vi "regulator1.vi"(0 "histereza":dbl, 4 "H2 [cm]":dbl, 5 "H1 [cm]":dbl, 6 "h2max":dbl, 7 "h2min":dbl, 8 "h1max":dbl, 9 "h1min":dbl) -> (1 "Zawor2":bool, 2 "Zawor1":bool, 3 "Pompa":bool)   [LabVIEW 2020]
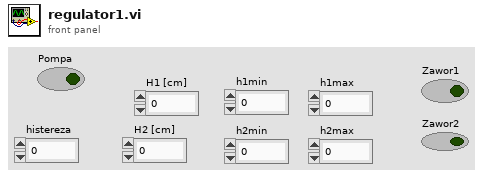
[diagram p1: front panel]
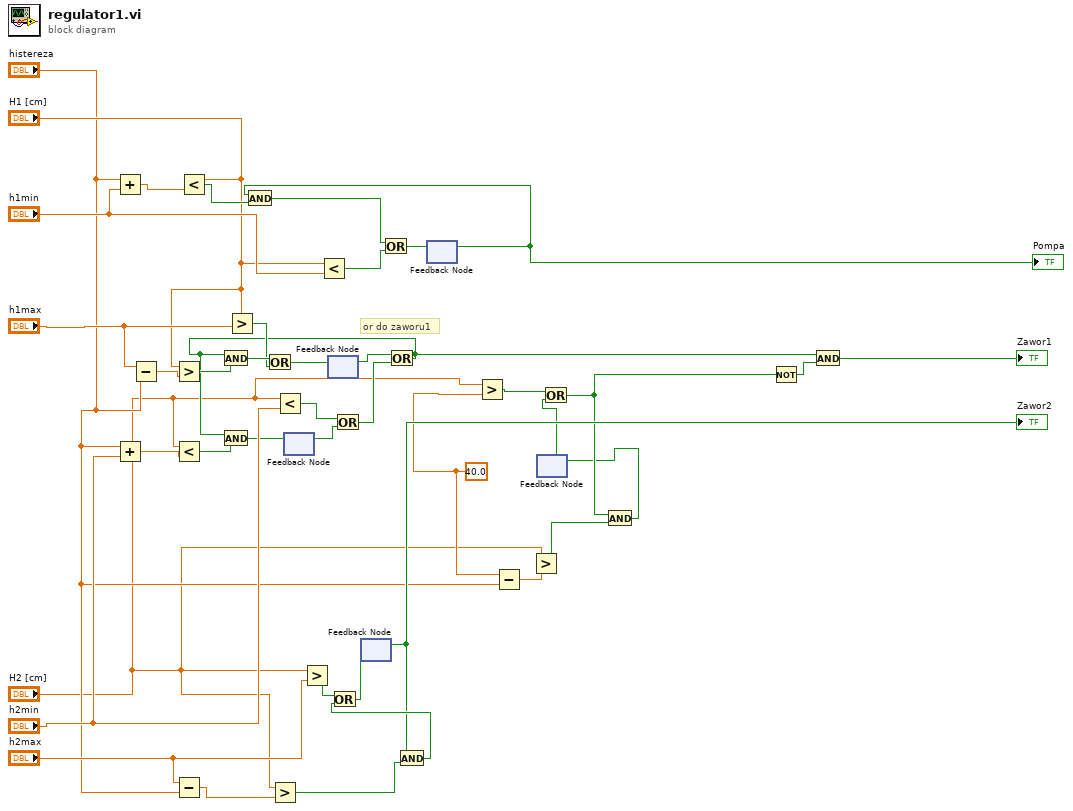
[diagram p0: block diagram]
diagram:
  w9 = 40.0
  # "or do zaworu1"
  n1 = Add(x="histereza", y="h1min") -> (x+y=w36:dbl)
  n2 = Add(x="histereza", y="h2min") -> (x+y=w22:dbl)
  n3 = Subtract(x="h1max", y="histereza") -> (x-y=w29:dbl)
  n4 = Greater?(x="H1 [cm]", y=w29) -> (0:w28:bool)
  n5 = Less?(x="H2 [cm]", y=w22) -> (x < y?=w24:bool)
  n6 = Subtract(x="h2max", y="histereza") -> (x-y=w18:dbl)
  n7 = Less?(x="H1 [cm]", y=w36) -> (x < y?=w35:bool)
  n8 = Greater?(x="H1 [cm]", y="h1max") -> (0:w32:bool)
  n9 = Greater?(x="H2 [cm]", y=w18) -> (0:w17:bool)
  n10 = Less?(x="H2 [cm]", y="h2min") -> (x < y?=w31:bool)
  n11 = feedback #1() -> (w20:bool)  [unwired: 1 in]
  n12 = Greater?(x="H2 [cm]", y="h2max") -> (0:w15:bool)
  n13 = Less?(x="H1 [cm]", y="h1min") -> (x < y?=w40:bool)
  n14 = feedback #2() -> (w26:bool)  [unwired: 1 in]
  n15 = Or(x=w31, y=w20) -> (x .or. y?=w30:bool)
  n16 = feedback #3() -> (w13:bool)  [unwired: 1 in]
  "Zawor2" <- w13
  n17 = Or(x=w26, y=w30) -> (x .or. y?=w12:bool)
  n18 = And(x=w12, y=w28) -> (x .and. y?=w33:bool)
  n19 = And(x=w12, y=w24) -> (x .and. y?=w21:bool)
  n20 = Or(x=w33, y=w32) -> (x .or. y?=w27:bool)
  n21 = feedback-in #1(w21) -> ()
  n22 = feedback-in #2(w27) -> ()
  n23 = And(x=w13, y=w17) -> (x .and. y?=w16:bool)
  n24 = Or(x=w15, y=w16) -> (x .or. y?=w14:bool)
  n25 = feedback-in #3(w14) -> ()
  n26 = feedback #4() -> (w38:bool)  [unwired: 1 in]
  "Pompa" <- w38
  n27 = And(x=w38, y=w35) -> (x .and. y?=w41:bool)
  n28 = Or(x=w41, y=w40) -> (x .or. y?=w39:bool)
  n29 = feedback-in #4(w39) -> ()
  n30 = Greater?(x="H2 [cm]", y=w9) -> (0:w4:bool)
  n31 = Subtract(x=w9, y="histereza") -> (x-y=w6:dbl)
  n32 = Greater?(x="H2 [cm]", y=w6) -> (0:w5:bool)
  n33 = feedback #5() -> (w1:bool)  [unwired: 1 in]
  n34 = Or(x=w4, y=w1) -> (x .or. y?=w3:bool)
  n35 = And(x=w3, y=w5) -> (x .and. y?=w2:bool)
  n36 = feedback-in #5(w2) -> ()
  n37 = Not(x=w3) -> (.not. x?=w8:bool)
  n38 = And(x=w12, y=w8) -> (x .and. y?=→"Zawor1":bool)
